vi "user_copy.vi"(8 "error in (no error)":errorcluster, 10 "old user name in":string) -> (0 "error out":errorcluster, 1 "cancelled?":bool, 2 "new user name out":string)   [LabVIEW 2010]
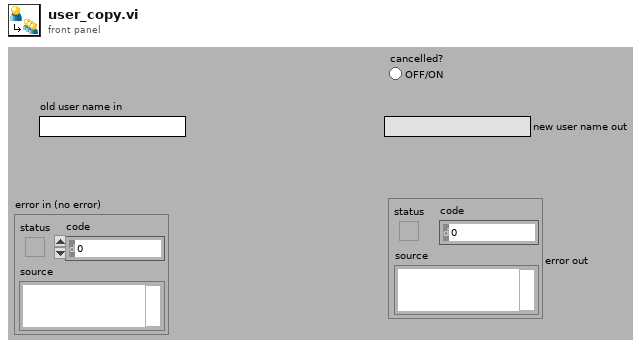
[diagram p1: front panel]
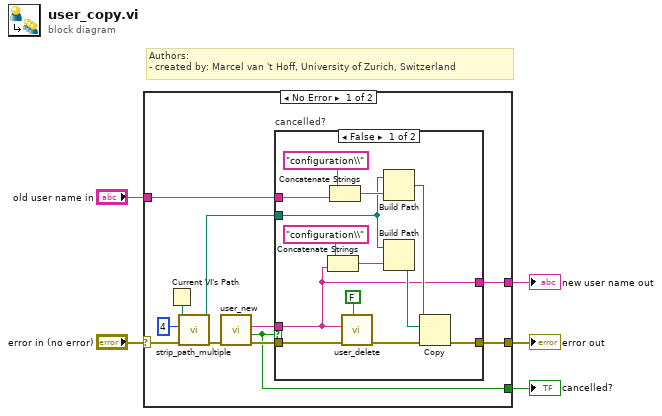
[diagram p0: block diagram]
diagram:
  # "Authors: \n- created by: Marcel van 't Hoff, University of Zurich, Switzerland"
  n1 = case shown="No Error" "error in (no error)" {
    selector: "error in (no error)" -> [w10 w32]
    tunnel: "old user name in" -> [w11 _]
    tunnel: [w9 w32] -> w3
    tunnel: [w7 _] -> w2
    tunnel: [w6 _] -> w1
    frame No Error {
      n2 = Current VI's Path() -> (path=w15:path)
      n3 = call "strip_path_multiple.vi"("error in (no error)"=w10, "number of strips"=4, "path in"=w15) -> ("error out"=w14:errorcluster, "path out"=w12:path)  [unwired: 7 in]
      n4 = call "user_new.vi"("error in (no error)"=w14) -> ("error IO"=w13:errorcluster, "cancelled?"=w6:bool, "user name out"=w8:string)  [unwired: 8 in]
      n5 = case "cancelled?" shown="False" w6 {
        tunnel: w13 -> [w27 w31]
        tunnel: w12 -> [w21 _]
        tunnel: w11 -> [w20 w30]
        tunnel: [w18 w31] -> w9
        tunnel: w8 -> [w17 _]
        tunnel: [w17 w30] -> w7
        frame False {
          n6 = Concatenate Strings("configuration\\" ("name or relative path"), w17) -> (w28:string)
          n7 = Concatenate Strings("configuration\\" ("name or relative path"), w20) -> (w23:string)
          n8 = call "user_delete.vi"("confirm deleting? (T)"=FALSE, "error in (no error)"=w27, "user name in"=w17) -> ("error out"=w24:errorcluster)  [unwired: 7 in, 1 out]
          n9 = Build Path(base path=w21, name or relative path=w23) -> (appended path=w19:path)
          n10 = Build Path(base path=w21, name or relative path=w28) -> (appended path=w25:path)
          n11 = Copy(8:w24, 10:w25, 11:w19) -> (0:w18:errorcluster)  [unwired: 2 in, 2 out]
        }
        frame True {
        }
      }
    }
    frame Error {
    }
  }
  "error out" <- w3
  "new user name out" <- w2
  "cancelled?" <- w1
